vi "reaction game.vi"() -> ()   [LabVIEW 2017]
panel:
  in  "stop":bool
  out "Result (ms)":dbl
  out "Message":string
  in  "Push Button":bool
  out "Indicator":bool
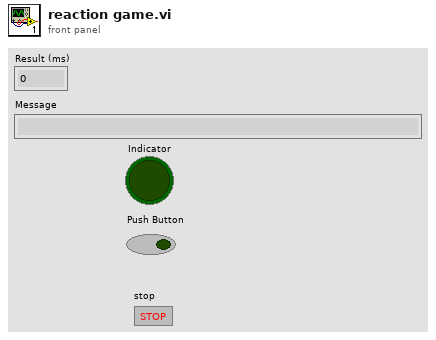
[diagram p1: front panel]
types:
  T1 = enum16{"BeginGame", "RandomWait", "WaitForReaction", "Calculate"}
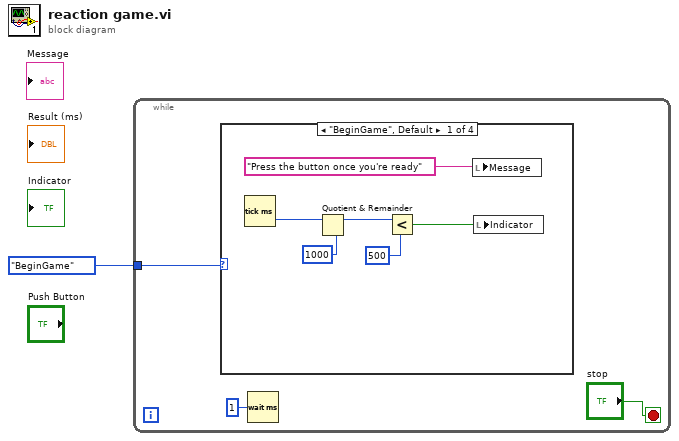
[diagram p0: block diagram]
diagram:
  n1 = while {
    tunnel: T1."BeginGame" -> [w2]
    stop <- "stop" stop-if-true
    n2 = case shown="\"BeginGame\", Default" w2 {
      frame "BeginGame", Default {
        n3 = Tick Count (ms)() -> (millisecond timer value=w9:u32)
        n4 = Quotient & Remainder(x=w9, y=u32 1000) -> (x-y*floor(x/y)=w7:u32)  [unwired: 1 out]
        n5 = Less?(x=w7, y=u32 500) -> (x < y?=w5:bool)
        n6 = local write "Message"("Press the button once you're ready") -> ()
        n7 = local write "Indicator"(w5) -> ()
      }
      frame "RandomWait" {
      }
      frame "WaitForReaction" {
      }
      frame "Calculate" {
      }
    }
    n8 = Wait (ms)(milliseconds to wait=u32 1) -> ()  [unwired: 1 out]
  }
